vi "svl_Auto Threshold.vi"(8 "error in (no error)":errorcluster, 9 "peak search settings":T2 {"threshold" format="%.2f"}, 11 "spectrum":T1 {"magnitude" format="%.2f"; "df [Hz]" format="%.2f"; "f0" format="%.2f"}) -> (0 "error out":errorcluster, 1 "peak search settings":T3 {"Threshold" format="%.2f"}, 3 "spectrum":cluster{"f0":dbl, "df":dbl, "spectrum":dbl[]} {"spectrum" format="%.2f"; "df" format="%.2f"; "f0" format="%.2f"})   [LabVIEW 2017]
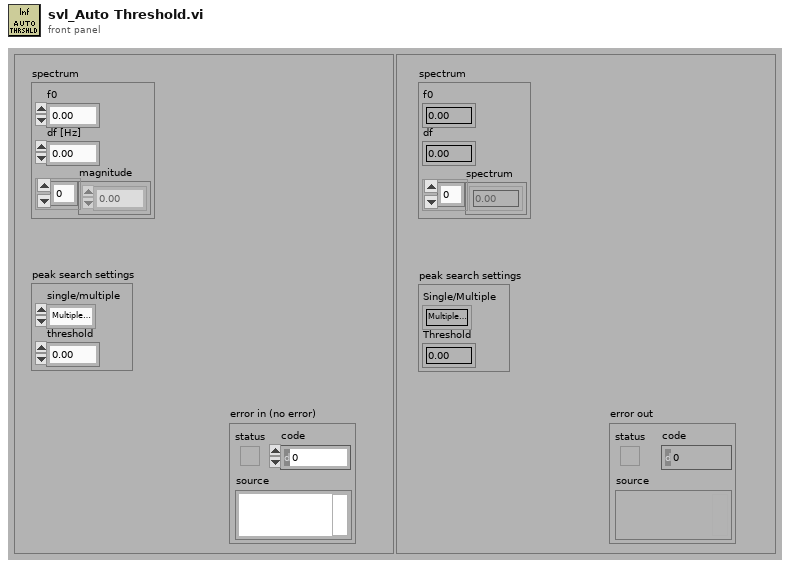
[diagram p1: front panel]
types:
  T1 = cluster{"f0":dbl, "df [Hz]":dbl, "magnitude":dbl[]}
  T2 = cluster{"single/multiple":enum16{"Multiple Peaks", "Single Max Peak"}, "threshold":dbl}
  T3 = cluster{"Single/Multiple":enum16{"Multiple Peaks", "Single Max Peak"}, "Threshold":dbl}
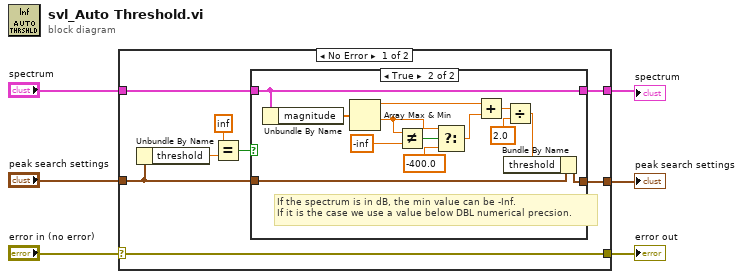
[diagram p0: block diagram]
diagram:
  n1 = case shown="No Error" "error in (no error)" {
    selector: "error in (no error)" -> [w7 w30]
    tunnel: [w14 w32] -> w6
    tunnel: [w13 w31] -> w5
    tunnel: "peak search settings" -> [w12 w31]
    tunnel: "spectrum" -> [w10 w32]
    tunnel: [w7 w30] -> w1
    frame No Error {
      n2 = Unbundle By Name(w12) -> ("threshold"=w9:dbl)
      n3 = Equal?(x=inf ("y"), y=w9) -> (x = y?=w11:bool)
      n4 = case shown="True" w11 {
        tunnel: w10 -> [w16 w27]
        tunnel: w12 -> [w15 w29]
        tunnel: [w15 w28] -> w13
        tunnel: [w16 w27] -> w14
        frame False {
        }
        frame True {
          # "If the spectrum is in dB, the min value can be -Inf.\nIf it is the case we use a value below DBL numerical precsion."
          n5 = Unbundle By Name(w27) -> ("magnitude"=w26:dbl[])
          n6 = Array Max & Min(array=w26) -> (max value=w25:dbl, min value=w19:dbl)  [unwired: 2 out]
          n7 = Not Equal?(x=w19, y=-inf) -> (x != y?=w21:bool)
          n8 = Select(t=w19, s=w21, f=-400.0 ("y")) -> (s? t:f=w18:dbl)
          n9 = Add(x=w25, y=w18) -> (x+y=w24:dbl)
          n10 = Divide(x=w24, y=2.0) -> (x/y=w22:dbl)
          n11 = Bundle By Name(cluster=w29, "threshold"=w22) -> (w28:T2)
        }
      }
    }
    frame Error {
    }
  }
  "spectrum" <- w6
  "peak search settings" <- w5
  "error out" <- w1
